vi "shuffle_ID_sequence.vi"(10 "sequence IDs with spaces":string) -> (2 "shuffled IDs":string)   [LabVIEW 2010, in "StimulatorAK101022TCP.lvclass"]
uses:
  StimulatorAK101022TCP.lvclass
  <vilib>/gmath/statdist.llb/Random Permutation.vi
  <vilib>/gmath/NI_Gmath.lvlib
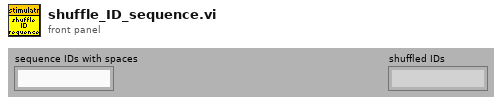
[diagram p1: front panel]
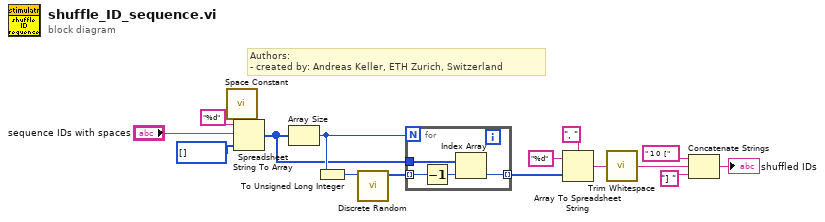
[diagram p0: block diagram]
diagram:
  # "Authors: \n- created by: Andreas Keller, ETH Zurich, Switzerland"
  n1 = call <vilib>:"Space Constant.vi"() -> ("String"=w16:string)
  n2 = Spreadsheet String To Array(delimiter (Tab)=w16, format string="%d", spreadsheet string="sequence IDs with spaces", array type (2D Dbl)=u32[] []) -> (array=w9:u32[])
  n3 = Array Size(array=w9) -> (size(s)=w11:i32)
  n4 = To Unsigned Long Integer(number=w11) -> (unsigned 32bit integer=w12:u32)
  n5 = call-poly <vilib>:"Discrete Random.vi"("N"=w12) -> ("random permutation"=w10:i32[])  [unwired: 9 in, 1 out]
  n6 = for {
    N: w11 -> [_]
    tunnel: w10 -> [w20] mode=indexing
    tunnel: w9 -> [w18]
    tunnel: [w17] -> w8 mode=indexing
    n7 = Decrement(x=w20) -> (x-1=w19:i32)
    n8 = Index Array(array=w18, index=w19) -> (element=w17:u32)
  }
  n9 = Array To Spreadsheet String(delimiter (Tab)=", ", array=w8, 3:"%d" ("format string")) -> (spreadsheet string=w5:string)
  n10 = call <vilib>:"Trim Whitespace.vi"("string"=w5) -> ("trimmed string"=w4:string)  [unwired: 1 in]
  n11 = Concatenate Strings(" 1 0  [" ("string"), w4, "] " ("string")) -> (→"shuffled IDs":string)
